vi "Clone and Condition Reference Waveform.vi"(0 "Reference Waveform":T1 {"Runtime Scaling" format="%#_6p"; "Sample Rate" format="%#_6p"; "Burst Length (s)" format="%#_6p"; "PAPR (dB)" format="%.2f"; "Signal Bandwidth (Hz)" format="%#_6p"}, 11 "error in (no error)":errorcluster) -> (4 "Conditioned Reference Waveform":T1 {"Runtime Scaling" format="%#_6p"; "Sample Rate" format="%#_6p"; "Burst Length (s)" format="%#_6p"; "PAPR (dB)" format="%.2f"; "Signal Bandwidth (Hz)" format="%#_6p"}, 15 "error out":errorcluster)   [LabVIEW 2019, in "Envelope Tracking.lvlib"]
doc: "Duplicates <b>Reference Waveform</b>, updates the name, and sets appropriate values for the waveform."
uses:
  Envelope Tracking.lvlib
  Common/Waveform.ctl
  Common/Common.lvlib
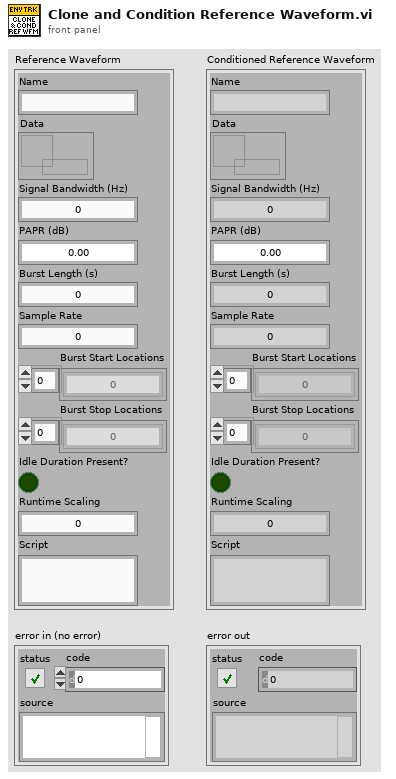
[diagram p1: front panel]
types:
  T1 = typedef "Common.lvlib/Waveform.ctl" = cluster{"Name":string, "Data":refnum<data-value>, "Signal Bandwidth (Hz)":dbl, "PAPR (dB)":dbl, "Burst Length (s)":dbl, "Sample Rate":dbl, "Burst Start Locations":i32[], "Burst Stop Locations":i32[], "Idle Duration Present?":bool, "Runtime Scaling":dbl, "Script":string}
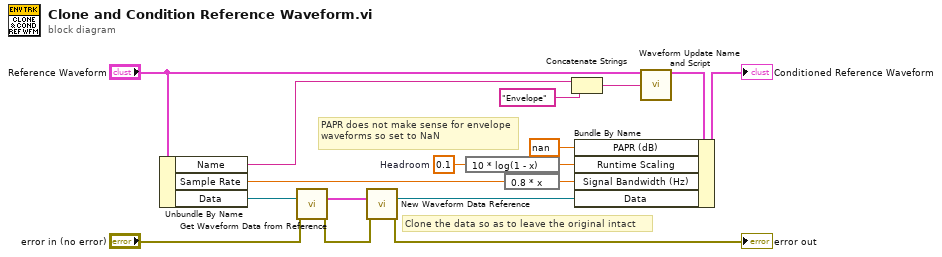
[diagram p0: block diagram]
diagram:
  w11 = 0.1  # Headroom
  # "Clone the data so as to leave the original intact"
  # "PAPR does not make sense for envelope waveforms so set to NaN"
  n1 = Unbundle By Name("Reference Waveform") -> ("Name"=w16:string, "Sample Rate"=w13:dbl, "Data"=w9:refnum<data-value>)
  n2 = call "Get Waveform Data from Reference.vi"("Waveform Data Reference"=w9, "error in (no error)"="error in (no error)") -> ("Waveform Data"=w8:cluster{"t0":dbl, "dt":dbl, "y":csg[]}, "error out"=w7:errorcluster)  [unwired: 12 in]
  n3 = call "New Waveform Data Reference.vi"("Waveform Data"=w8, "error in (no error)"=w7) -> ("Waveform Data Reference"=w6:refnum<data-value>, "error out"=→"error out":errorcluster)  [unwired: 12 in]
  n4 = expression code="10 * log(1 - x)"(w11) -> (w5:dbl)
  n5 = expression code="0.8 * x"(w13) -> (w12:dbl)
  n6 = Concatenate Strings(w16, "Envelope" ("string")) -> (w15:string)
  n7 = call "Waveform Update Name and Script.vi"("Waveform in"="Reference Waveform", "New Waveform Name"=w15) -> ("Waveform out"=w14:T1)  [unwired: 13 in]
  n8 = Bundle By Name(cluster=w14, "PAPR (dB)"=nan, "Runtime Scaling"=w5, "Signal Bandwidth (Hz)"=w12, "Data"=w6) -> (→"Conditioned Reference Waveform":T1)
